vi "FindMessage.vi"(11 "Message in":string) -> (1 "found?":bool, 2 "Message":string, 3 "Remaining buffer":string)   [LabVIEW 2013, in "MixerMessage.lvclass"]
doc: "Parses and interpretes the input string. If a complete packet from the remote host is found, \"found?\" should return TRUE. In that the case, the response should contain the type and the message data in the variant. \nIf the found message is an acknowledgement to the \"Sent message in\", the isAck? boolean should return TRUE.\nAnything left in the Message in string after the first message has been found should be returned in Remaining buffer"
uses:
  MixerMessage.lvclass
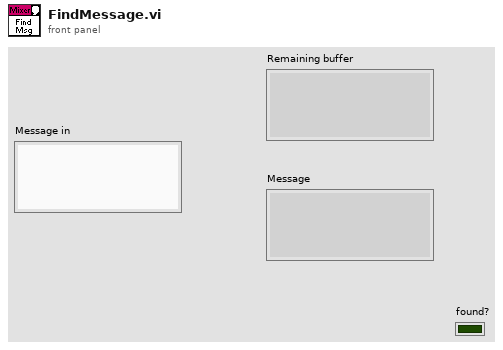
[diagram p1: front panel]
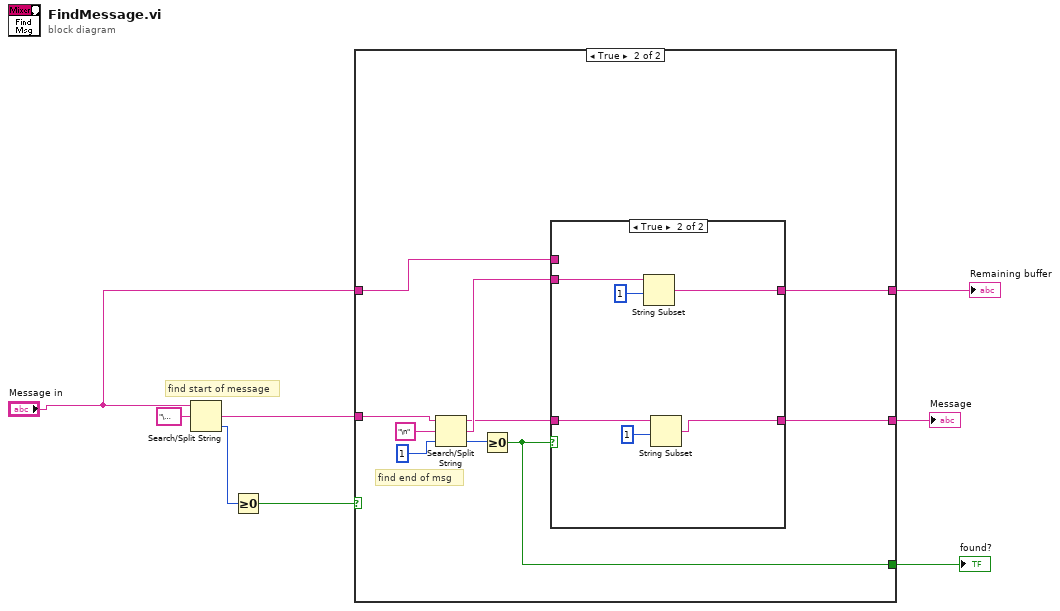
[diagram p0: block diagram]
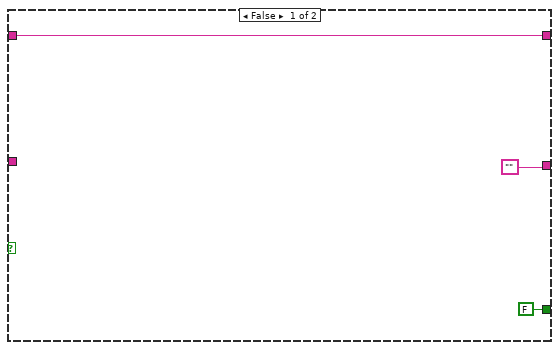
[diagram p2: hidden frame]
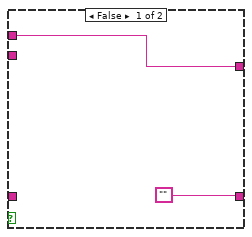
[diagram p3: hidden frame]
diagram:
  # "find start of message"
  n1 = Search/Split String(string="Message in", search string/char (-)="\u0002") -> (match + rest of string=w6:string, offset of match=w7:i32)  [unwired: 1 in, 1 out]
  n2 = Greater Or Equal To 0?(x=w7) -> (x >= 0?=w5:bool)
  n3 = case shown="True" w5 {
    tunnel: w6 -> [_ w18]
    tunnel: ["" w13] -> w4
    tunnel: [w11 w16] -> w2
    tunnel: [FALSE w14] -> w3
    tunnel: "Message in" -> [w11 w12]
    frame False {
    }
    frame True {
      # "find end of msg"
      n4 = Search/Split String(string=w18, search string/char (-)="\n", offset (0)=1) -> (substring before match=w15:string, match + rest of string=w17:string, offset of match=w20:i32)
      n5 = Greater Or Equal To 0?(x=w20) -> (x >= 0?=w14:bool)
      n6 = case shown="True" w14 {
        tunnel: w17 -> [_ w28]
        tunnel: [w23 w27] -> w16
        tunnel: w15 -> [_ w25]
        tunnel: ["" w24] -> w13
        tunnel: w12 -> [w23 _]
        frame False {
        }
        frame True {
          n7 = String Subset(string=w28, offset (0)=1) -> (substring=w27:string)  [unwired: 1 in]
          n8 = String Subset(string=w25, offset (0)=1) -> (substring=w24:string)  [unwired: 1 in]
        }
      }
    }
  }
  "found?" <- w3
  "Message" <- w4
  "Remaining buffer" <- w2
